vi "example use of turn power block.vi"(8 "error in (no error)":errorcluster, 10 "desired angle":dbl, 11 "RobotDriveDevRef":T1={"DevStatus"={"status"=FALSE, "code"=0, "source"=""}, "Motors[]"=[], "Square Inputs"=FALSE, "Max Output"=1.0}) -> (0 "error out":errorcluster, 3 "RobotDriveDevRef 2":T1={"DevStatus"={"status"=FALSE, "code"=0, "source"=""}, "Motors[]"=[], "Square Inputs"=FALSE, "Max Output"=1.0})   [LabVIEW 2016]
uses:
  <vilib>/Rock Robotics/WPI/RobotDrive/WPI_RobotDriveDevRef.ctl
  <vilib>/Rock Robotics/WPI/MotorControl/WPI_MotorControlDeviceRef.ctl
  <vilib>/Rock Robotics/WPI/MotorControl/WPI_MotorControlType.ctl
  <vilib>/Rock Robotics/SystemInterfaces/DIO/FPGA_DIOPWMChannel.ctl
  <vilib>/Rock Robotics/WPI/PWM/WPI_PWMDeadband.ctl
  Robot Global Data.vi
  <vilib>/Rock Robotics/WPI/RobotDrive/WPI_RobotDriveArcadeDrive_Standard(NoSaturation).vi
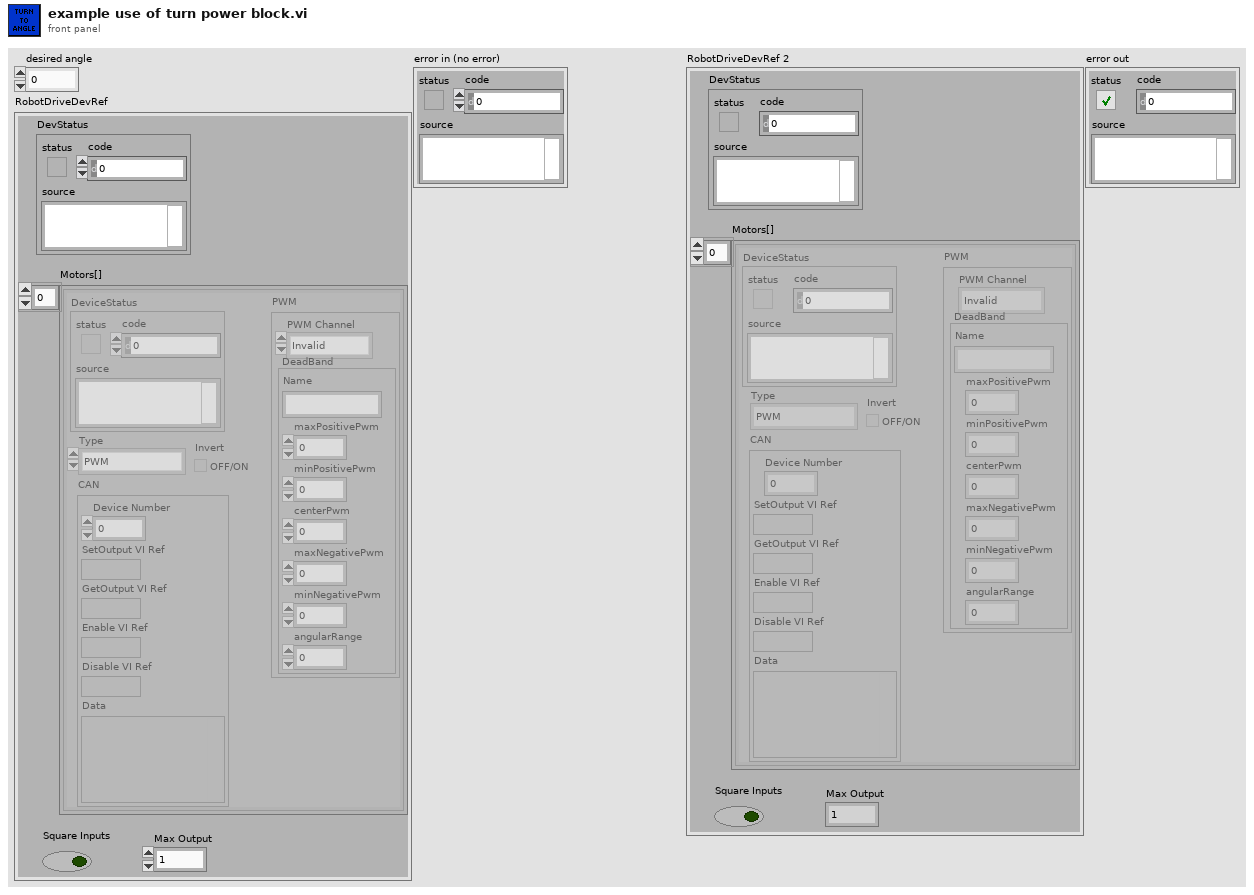
[diagram p1: front panel]
types:
  T1 = typedef "WPI_RobotDriveDevRef.ctl" = cluster{"DevStatus":errorcluster, "Motors[]":T2[], "Square Inputs":bool, "Max Output":dbl}
  T2 = typedef "WPI_MotorControlDeviceRef.ctl" = cluster{"DeviceStatus":errorcluster, "Type":T3, "PWM":cluster{"PWM Channel":T4, "DeadBand":T5}, "CAN":cluster{"Device Number":u8, "SetOutput VI Ref":variant, "GetOutput VI Ref":variant, "Enable VI Ref":variant, "Disable VI Ref":variant, "Data":variant}, "Invert":bool}
  T3 = typedef "WPI_MotorControlType.ctl" = enum16{"PWM", "CAN"}
  T4 = typedef "FPGA_DIOPWMChannel.ctl" = enum8{"PWM 0", "PWM 1", "PWM 2", "PWM 3", "PWM 4", "PWM 5", "PWM 6", "PWM 7", "PWM 8", "PWM 9", "PWM MXP 0", "PWM MXP 1", "PWM MXP 2", "PWM MXP 3", "PWM MXP 4", "PWM MXP 5", "PWM MXP 6", "PWM MXP 7", "PWM MXP 8", "PWM MXP 9", "Invalid"}
  T5 = typedef "WPI_PWMDeadband.ctl" = cluster{"Name":string, "maxPositivePwm":i32, "minPositivePwm":i32, "centerPwm":i32, "maxNegativePwm":i32, "minNegativePwm":i32, "angularRange":u16}
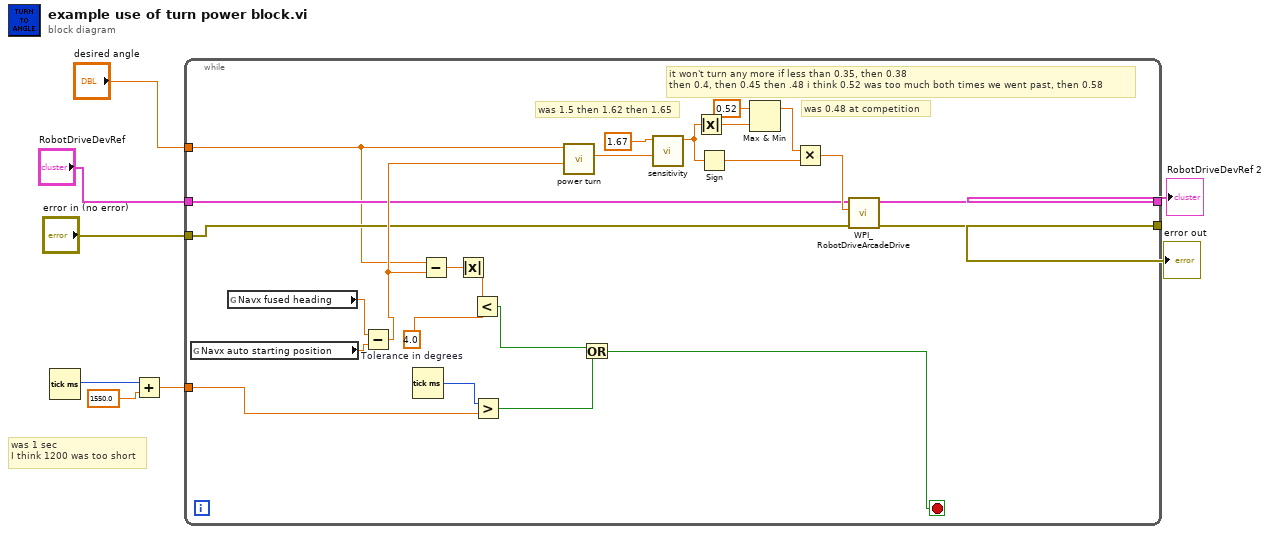
[diagram p0: block diagram]
diagram:
  # "was 1 sec\nI think 1200 was too short"
  n1 = Tick Count (ms)() -> (millisecond timer value=w8:u32)
  n2 = Add(x=w8, y=1550.0) -> (x+y=w1:dbl)
  n3 = while {
    tunnel: [w25] -> w6
    tunnel: [w24] -> w5
    tunnel: "RobotDriveDevRef" -> [w12]
    tunnel: "error in (no error)" -> [w11]
    tunnel: "desired angle" -> [w10]
    tunnel: w1 -> [w9]
    stop <- w26 stop-if-true
    w32 = 4.0  # Tolerance in degrees
    # "was 0.48 at competition"
    # "it won't turn any more if less than 0.35, then 0.38\nthen 0.4, then 0.45 then .48 i think 0.52 was too much both times we went past, then 0.58"
    # "was 1.5 then 1.62 then 1.65"
    n4 = global read "Robot Global Data.vi" "Navx auto starting position"() -> (w15:dbl)
    n5 = global read "Robot Global Data.vi" "Navx fused heading"() -> (w14:dbl)
    n6 = Subtract(x=w14, y=w15) -> (x-y=w13:dbl)
    n7 = Tick Count (ms)() -> (millisecond timer value=w29:u32)
    n8 = Subtract(x=w10, y=w13) -> (x-y=w30:dbl)
    n9 = Absolute Value(x=w30) -> (abs(x)=w31:dbl)
    n10 = Less?(x=w31, y=w32) -> (x < y?=w28:bool)
    n11 = Greater?(x=w29, y=w9) -> (0:w27:bool)
    n12 = call "power turn.vi"("current angle"=w13, "desired angle(degrees)"=w10) -> ("output"=w23:dbl)  [unwired: 9 in]
    n13 = Or(x=w28, y=w27) -> (x .or. y?=w26:bool)
    n14 = call "sensitivity.vi"("x"=w23, "sensitivity"=1.67) -> ("scaled value"=w21:dbl)  [unwired: 9 in]
    n15 = Absolute Value(x=w21) -> (abs(x)=w20:dbl)
    n16 = Sign(1:w21) -> (0:w17:dbl)
    n17 = Max & Min(x=0.52, y=w20) -> (max(x,y)=w18:dbl)  [unwired: 1 out]
    n18 = Multiply(x=w18, y=w17) -> (x*y=w16:dbl)
    n19 = call-poly <vilib>:"WPI_RobotDriveArcadeDrive.vi"("error in (no error)"=w11, "X axis value"=w16, "RobotDriveDevRef"=w12) -> ("error out"=w24:errorcluster, "RobotDriveDevRef"=w25:T1)  [unwired: 6 in, 1 out]
  }
  "RobotDriveDevRef 2" <- w6
  "error out" <- w5
